vi "mod_first iteration.vi"() -> (0 "First Iteration?: T/F":bool)   [LabVIEW 2020, in "niAMT.lvlib"]
uses:
  <vilib>/addons/Modulation/niAMT.lvlib
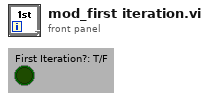
[diagram p1: front panel]
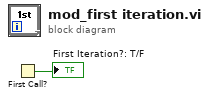
[diagram p0: block diagram]
diagram:
  n1 = First Call?() -> (First Call?: T/F=→"First Iteration?: T/F":bool)
